vi "Element_Order_Numbers.vi"(1 "Element_Array":variant[](array[variant]), 2 "Element":variant) -> (0 "Order_numbers":i32[](array[numeric]))   [LabVIEW 2019]
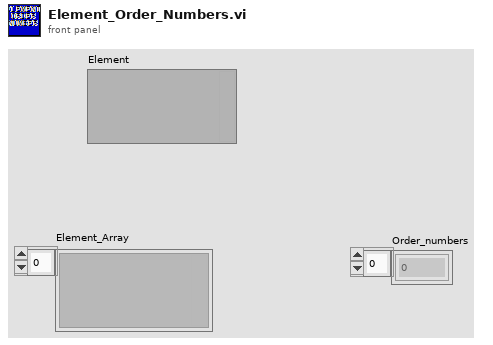
[diagram p1: front panel]
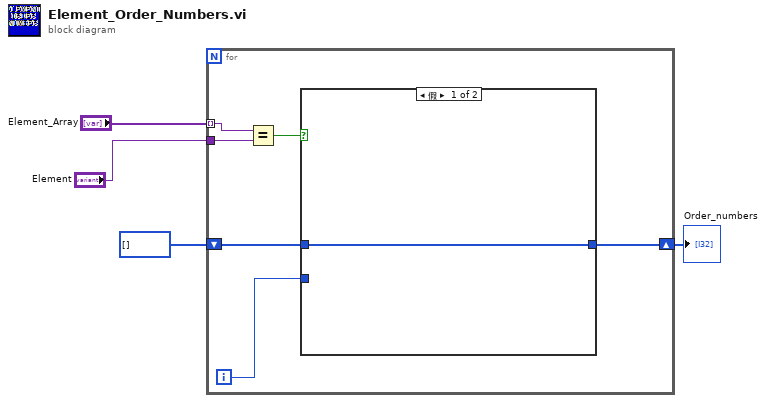
[diagram p0: block diagram]
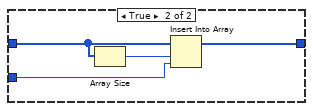
[diagram p2: hidden frame]
diagram:
  n1 = for {
    tunnel: "Element_Array" -> [w10] mode=indexing
    shift-right: [w6] -> w1
    shift-left: i32[] [] -> [w7]
    tunnel: "Element" -> [w9]
    i -> [w5]
    n2 = Equal?(x=w10, y=w9) -> (x = y?=w8:bool)
    n3 = case shown="假" w8 {
      tunnel: w7 -> [w11 w13]
      tunnel: [w11 w15] -> w6
      tunnel: w5 -> [_ w12]
      frame False {
      }
      frame True {
        n4 = Array Size(array=w13) -> (size(s)=w14:i32)
        n5 = Insert Into Array(array=w13, index=w14, new element=w12) -> (w15:i32[])
      }
    }
  }
  "Order_numbers" <- w1
